vi "Get All Processes.vi"(8 "error in (no error)":errorcluster, 11 "Application In":refnum<class "Application.lvclass">) -> (0 "error out":errorcluster, 2 "App Processes":refnum<class "Process.lvclass">[](array[class]), 3 "Application Out":refnum<class "Application.lvclass">)   [LabVIEW 2020, in "Application.lvclass"]
doc: "Get all processes owned by the application."
uses:
  Application.lvclass
  Application.lvclass/Application.ctl
  Process/Process.lvclass
  C:/git/astemes-triarc-framework/source/Framework/Process/Process.lvclass
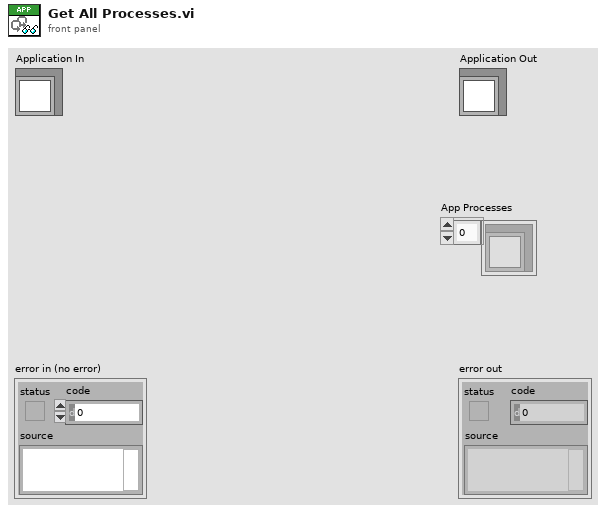
[diagram p1: front panel]
types:
  T1 = typedef "Process.lvclass/Lifecycle State.ctl" = enum16{"Uninitialized", "Initialized", "Started", "Running", "Stopped", "Finished"}
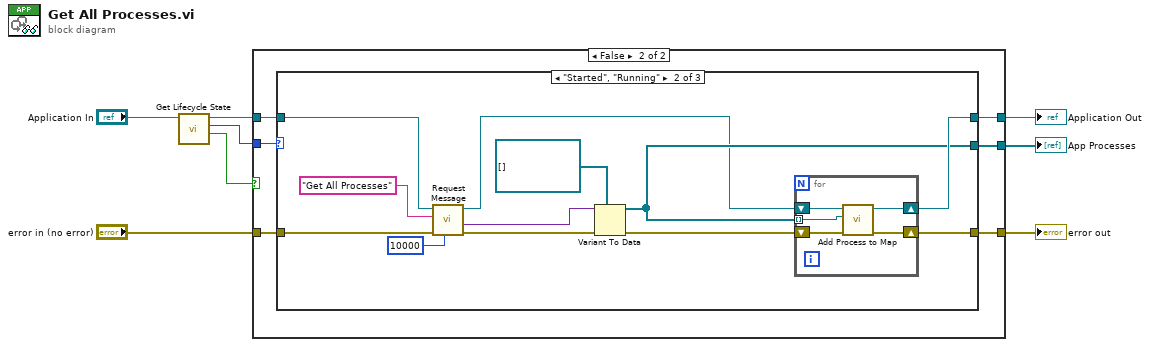
[diagram p0: block diagram]
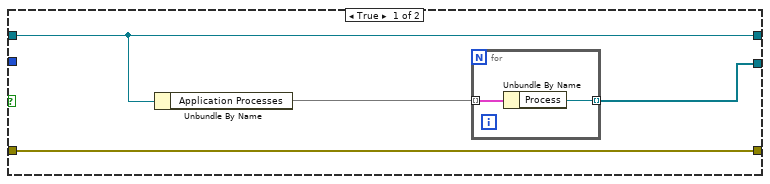
[diagram p2: hidden frame]
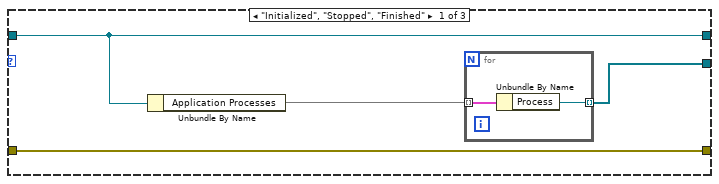
[diagram p3: hidden frame]
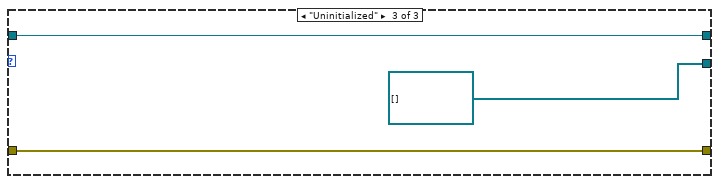
[diagram p4: hidden frame]
diagram:
  n1 = call "Get Lifecycle State.vi"("Process In"="Application In") -> ("In Process Loop?"=w3:bool, "Lifecycle State"=w2:T1, "Process Out"=w4:refnum<class "Application.lvclass">)  [unwired: 7 in, 1 out]
  n2 = case shown="False" w3 {
    tunnel: "error in (no error)" -> [w9 w20]
    tunnel: [w9 w16] -> w8
    tunnel: [w10 w17] -> w7
    tunnel: w4 -> [w11 w19]
    tunnel: [w11 w18] -> w5
    tunnel: w2 -> [_ w15]
    frame True {
      n3 = Unbundle By Name(w11) -> ("Application Processes"=w12:map{string, refnum<class "Process.lvclass">})
      n4 = for {
        tunnel: [w13] -> w10 mode=indexing
        tunnel: w12 -> [w14] mode=indexing
        n5 = Unbundle By Name(w14) -> ("Process"=w13:refnum<class "Process.lvclass">)
      }
    }
    frame False {
      n6 = case shown="\"Started\", \"Running\"" w15 {
        tunnel: w20 -> [w23 w38 w44]
        tunnel: w19 -> [w21 w34 w46]
        tunnel: [w21 w31 w46] -> w18
        tunnel: [w22 w30 refnum<class "Process.lvclass">[] [] ("Rig Process")] -> w17
        tunnel: [w23 w27 w44] -> w16
        frame "Initialized", "Stopped", "Finished" {
          n7 = Unbundle By Name(w21) -> ("Application Processes"=w24:map{string, refnum<class "Process.lvclass">})
          n8 = for {
            tunnel: [w25] -> w22 mode=indexing
            tunnel: w24 -> [w26] mode=indexing
            n9 = Unbundle By Name(w26) -> ("Process"=w25:refnum<class "Process.lvclass">)
          }
        }
        frame "Started", "Running" {
          n10 = call "Request Message.vi"("timeout in ms (-1)"=10000, "error in (no error)"=w38, "Request Message"="Get All Processes", "Process In"=w34) -> ("error out"=w37:errorcluster, "Response Message Data"=w35:variant, "Process Out"=w29:refnum<class "Application.lvclass">)  [unwired: 3 in, 2 out]
          n11 = Variant To Data(error in=w37, type=refnum<class "Process.lvclass">[] [] ("Rig Process"), Variant=w35) -> (data=w30:refnum<class "Process.lvclass">[], error out=w28:errorcluster)
          n12 = for {
            tunnel: w30 -> [w42] mode=indexing
            shift-right: [w41] -> w31
            shift-left: w29 -> [w43]
            shift-right: [w39] -> w27
            shift-left: w28 -> [w40]
            n13 = call "Add Process to Map.vi"("error in (no error)"=w40, "Process Out"=w42, "Application In"=w43) -> ("error out"=w39:errorcluster, "Application Out"=w41:refnum<class "Application.lvclass">)  [unwired: 7 in]
          }
        }
        frame "Uninitialized" {
        }
      }
    }
  }
  "error out" <- w8
  "Application Out" <- w5
  "App Processes" <- w7
